vi "Boiler.vi"() -> ()   [LabVIEW 2014]
uses:
  Controls/Boiler Controls.ctl
  Controls/Boiler Simulation Controls.ctl
  Controls/Boiler Status Indicators.ctl
  Controls/Boiler state enum.ctl
  Controls/Boiler runtime status indicators.ctl
  Controls/Log file FGV action enum.ctl
  Controls/Log event enum.ctl
panel:
  in  "stop":bool
  out "Boiler Status Indicators":T1 {"Time Count" format="%.2g"}
  in  "Boiler Simulation Controls":T2 {"Flame Sensor Value (%)" min=0.0 max=100.0 scale=0.0..100.0}
  in  "Boiler Controls":T3 {"Fuel Valve Position" min=0.0 max=100.0 scale=0.0..100.0 scale format="%.2f"}
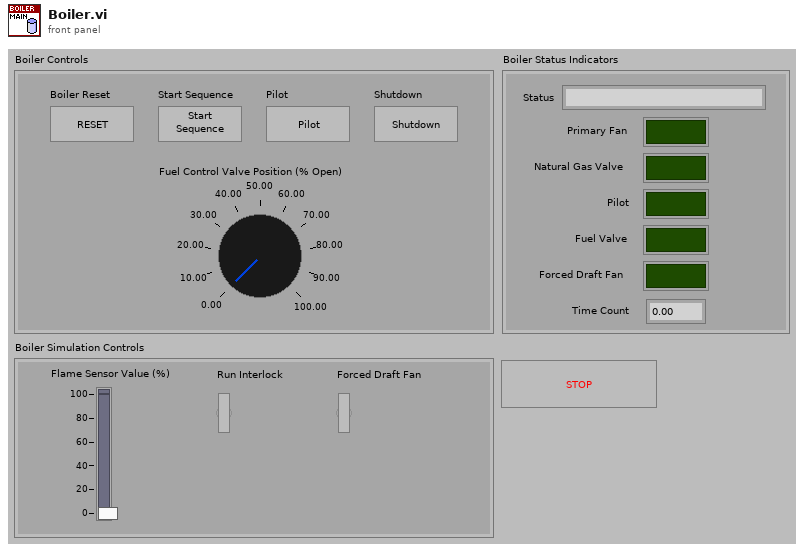
[diagram p1: front panel]
types:
  T1 = typedef "Boiler Status Indicators.ctl" = cluster{"Status":string, "Primary Fan":bool, "Natural Gas Valve":bool, "Pilot":bool, "Fuel Valve":bool, "Forced Draft Fan":bool, "Time Count":dbl}
  T2 = typedef "Boiler Simulation Controls.ctl" = cluster{"Flame Sensor Value (%)":dbl, "Run Interlock":bool, "Forced Draft Fan":bool}
  T3 = typedef "Boiler Controls.ctl" = cluster{"Boiler Reset":bool, "Start Sequence":bool, "Pilot":bool, "Shutdown":bool, "Fuel Valve Position":dbl}
  T4 = typedef "Boiler state enum.ctl" = enum16{"Initialize", "Wait on user action", "Start", "Pre-purge (running)", "Pre-purge (complete)", "Ignition (Ignite Pilot)", "Prove The Pilot", "Boiler Running", "Shutdown and Purge", "End"}
  T5 = typedef "Log file FGV action enum.ctl" = enum16{"open log file", "log event", "close log file"}
  T6 = typedef "Log event enum.ctl" = enum16{"Boiler Initialized", "Boiler Ready", "Start Pre-Purge", "Pre-Purge Complete", "Pilot ON", "Pilot proved", "Forced Draft Fan ON", "Boiler Running", "Start Shutdown Purge", "Shutdown Purge Complete"}
  T7 = typedef "Boiler runtime status indicators.ctl" = cluster{"Pre purge ready":bool, "Pre-purge complete":bool, "Pre-purge running":bool, "Pilot ignition running":bool, "Boiler Running":bool, "Shutdown running":bool, "Pilot proved":bool, "start time (ms)":u32}
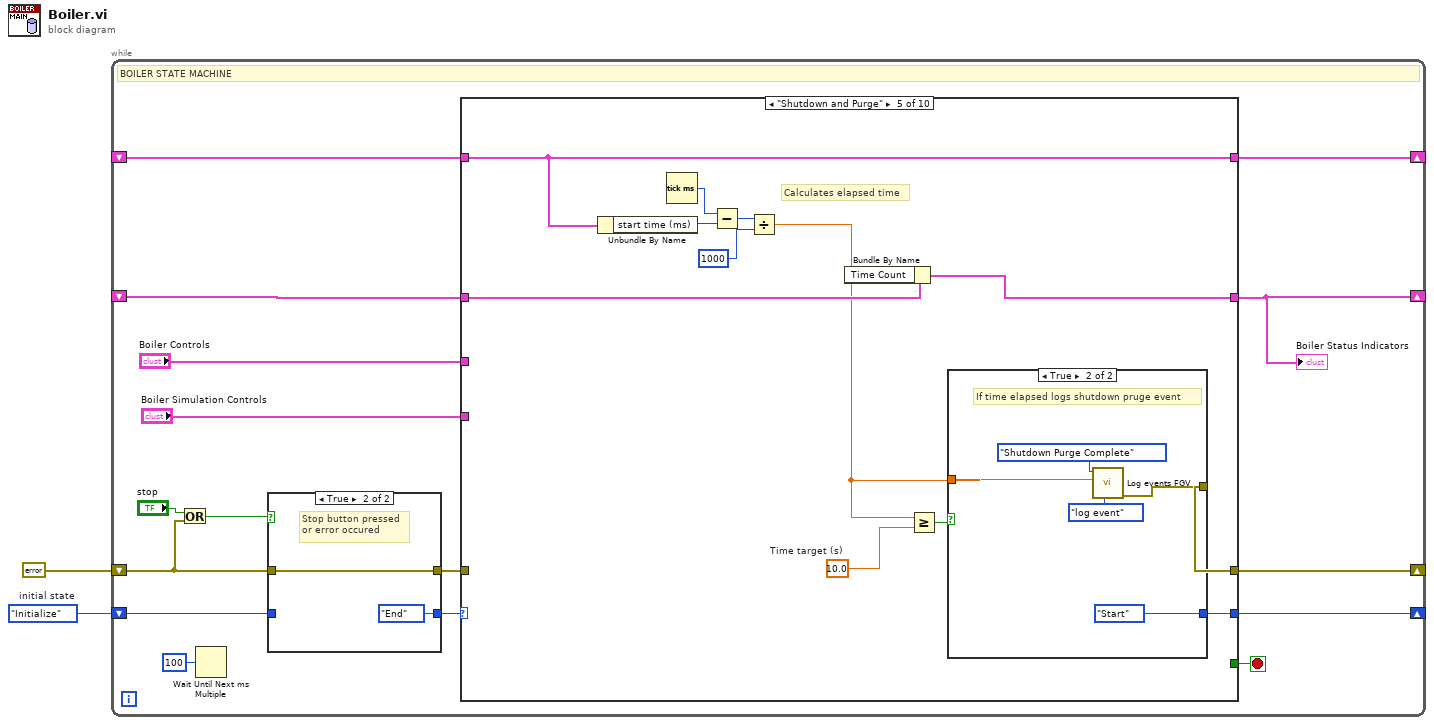
[diagram p0: block diagram]
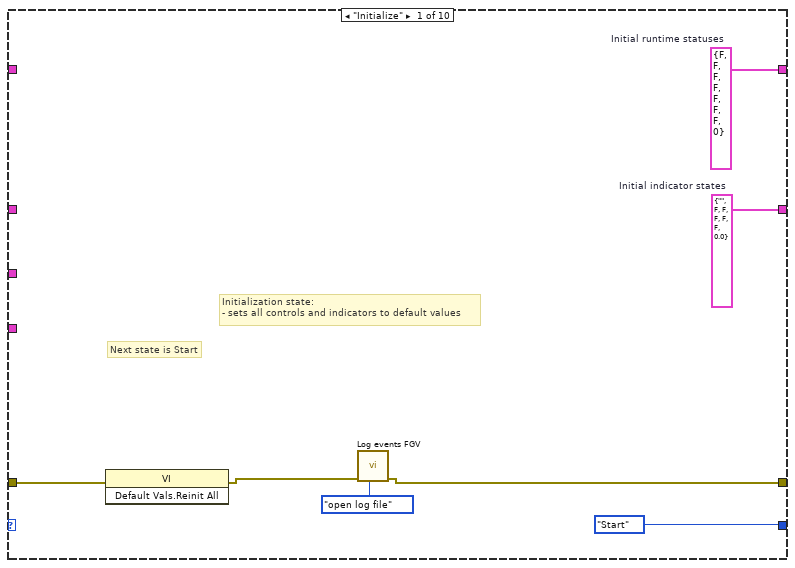
[diagram p3: hidden frame]
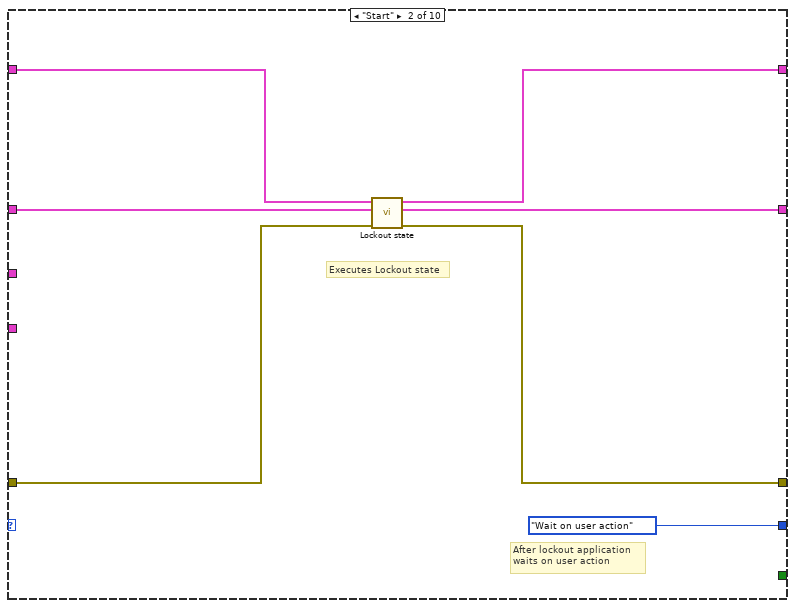
[diagram p4: hidden frame]
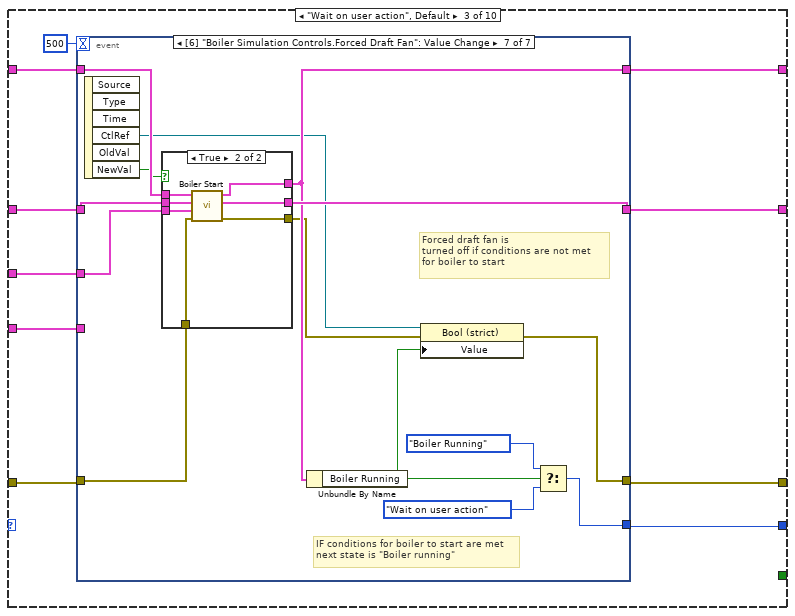
[diagram p5: hidden frame]
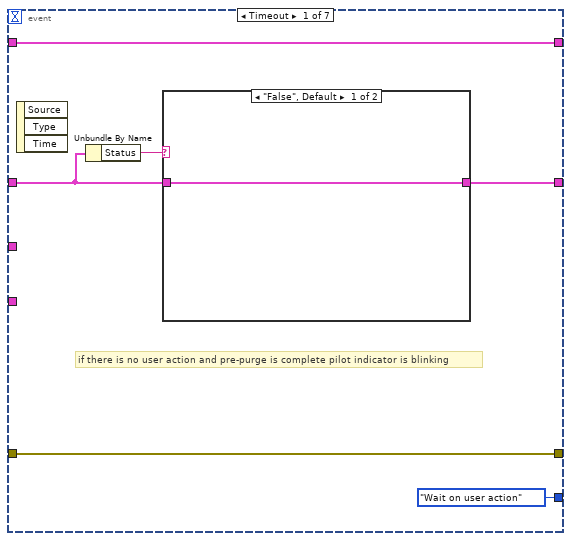
[diagram p6: hidden frame]
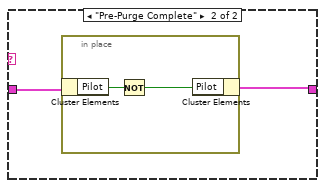
[diagram p7: hidden frame]
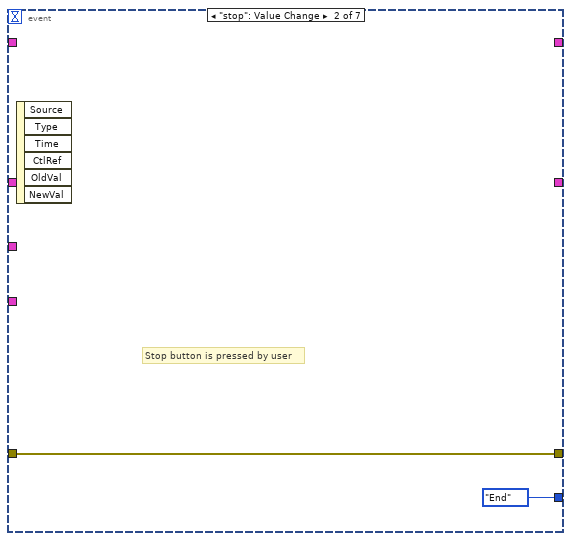
[diagram p8: hidden frame]
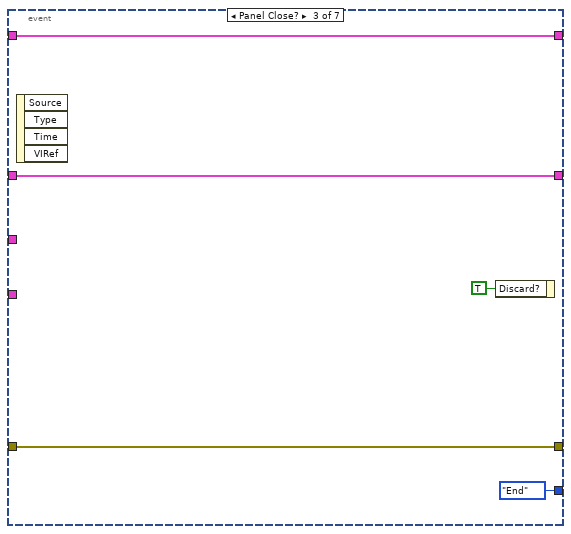
[diagram p9: hidden frame]
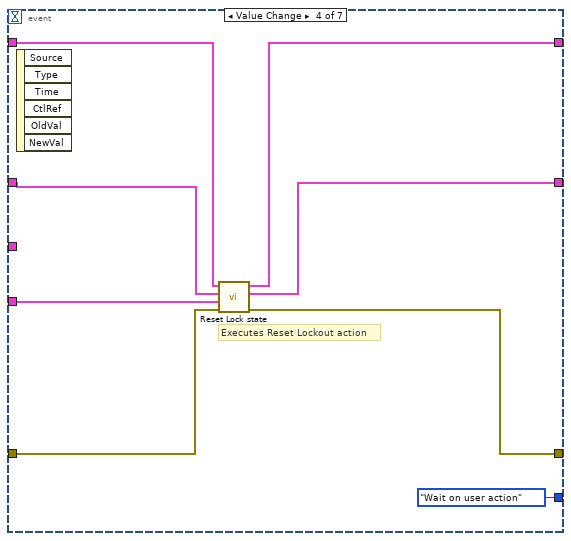
[diagram p10: hidden frame]
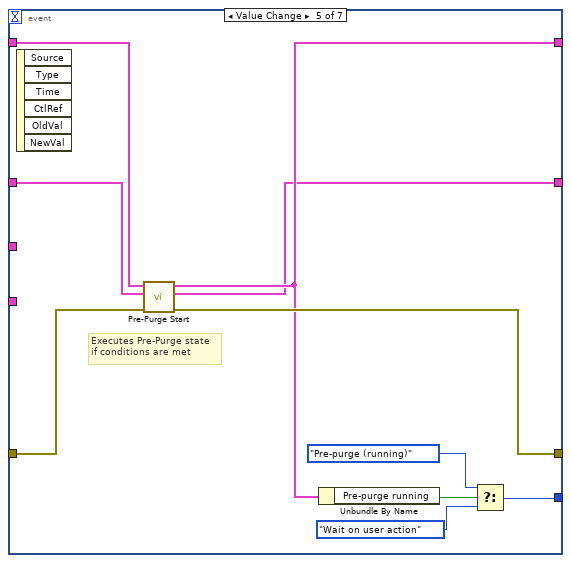
[diagram p11: hidden frame]
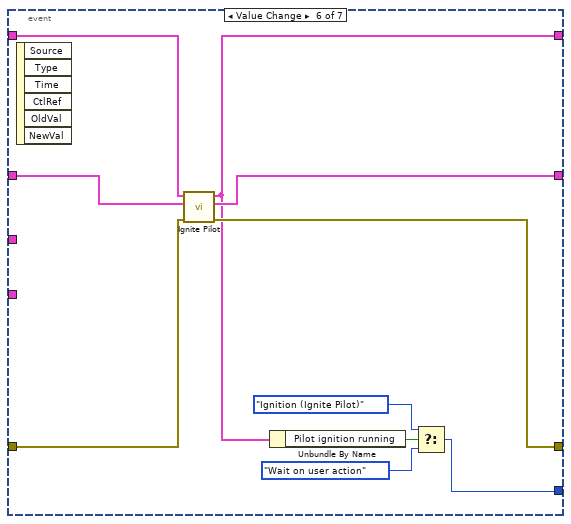
[diagram p12: hidden frame]
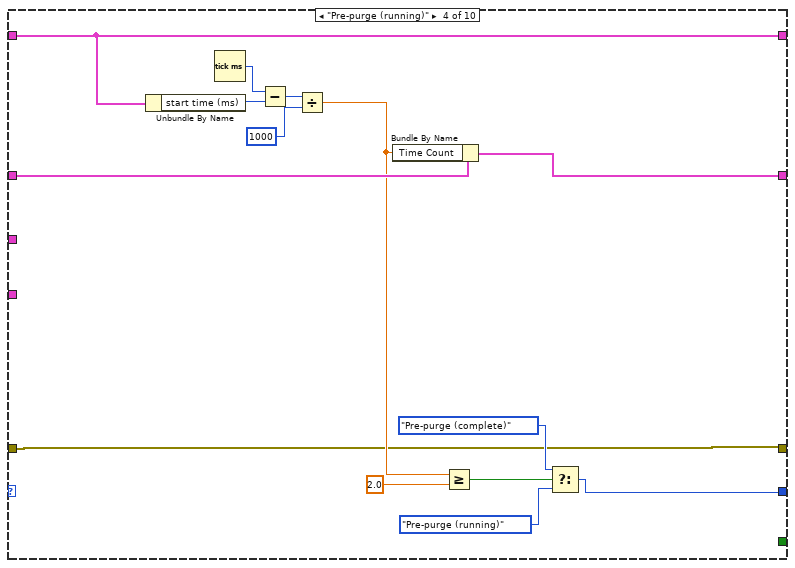
[diagram p14: hidden frame]
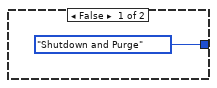
[diagram p15: hidden frame]
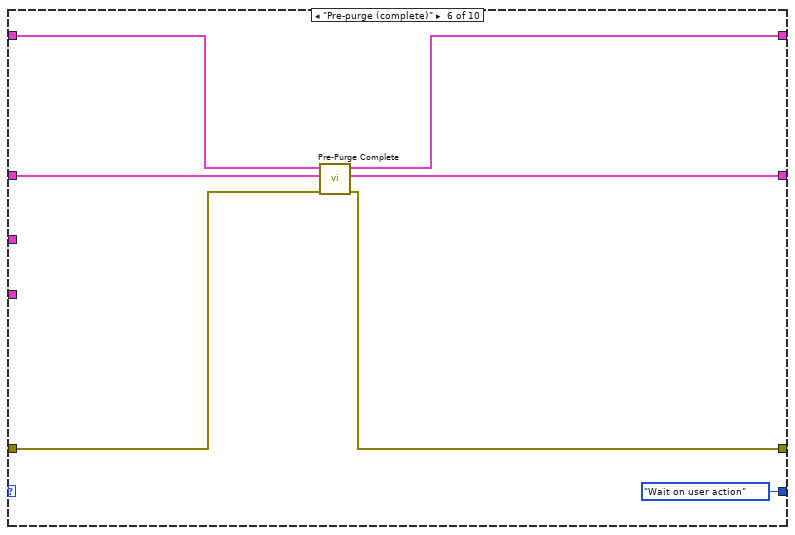
[diagram p16: hidden frame]
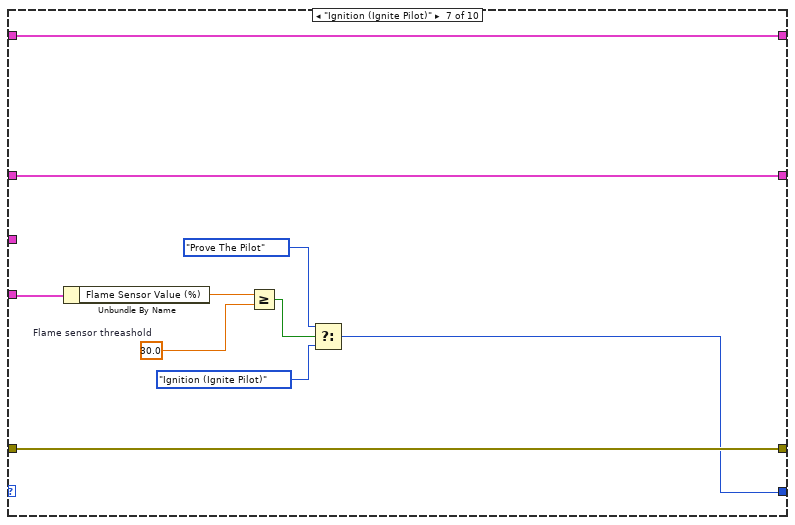
[diagram p17: hidden frame]
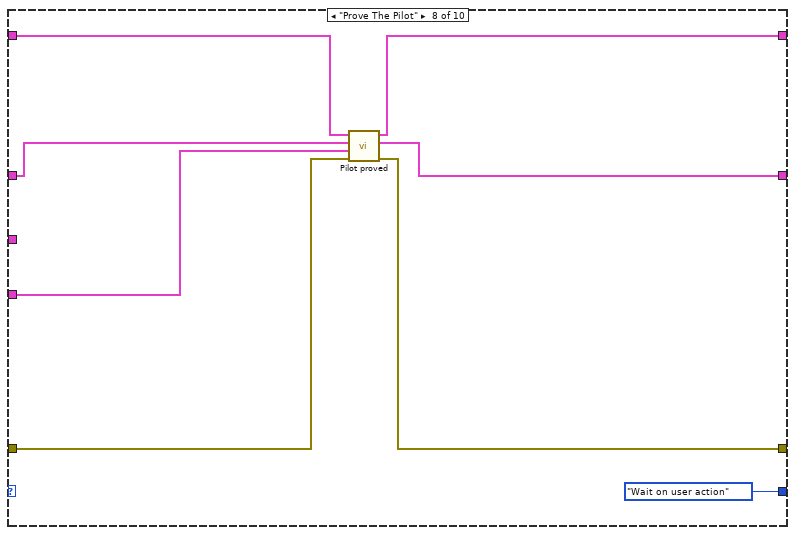
[diagram p18: hidden frame]
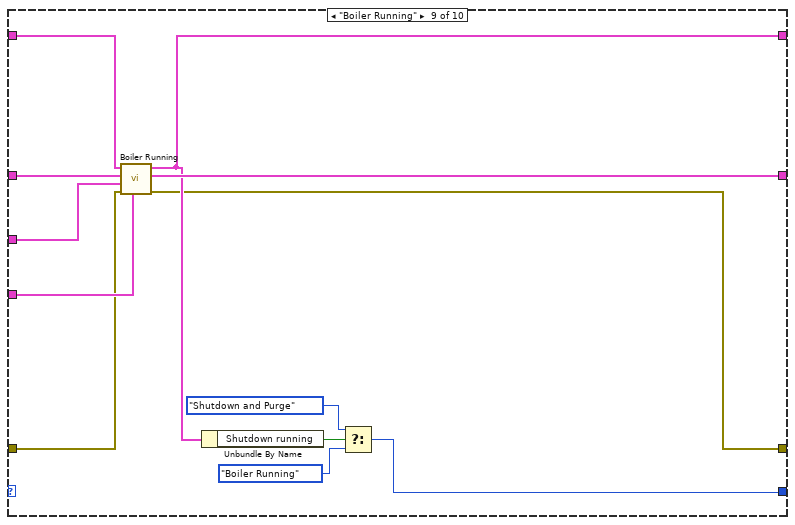
[diagram p19: hidden frame]
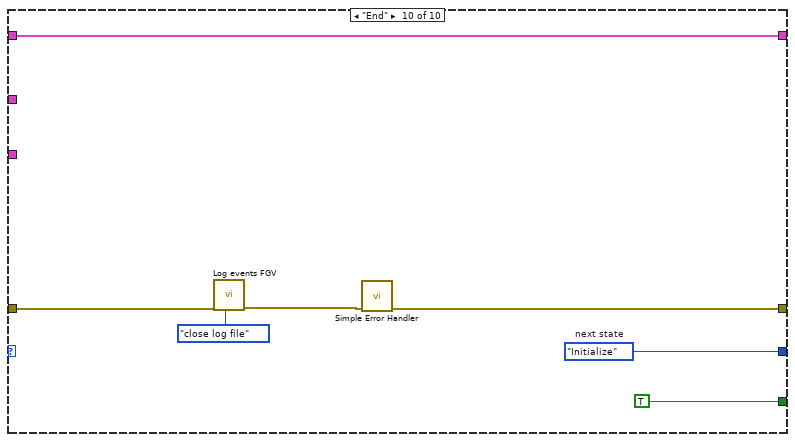
[diagram p20: hidden frame]
diagram:
  w2 = Boiler_state_enum."Initialize"  # initial state
  n1 = while {
    shift-right: [w8] -> _
    shift-left: w2 -> [w13]
    shift-right: [w17] -> _
    shift-left: _ -> [w18]
    shift-right: [w10] -> _
    shift-left: errorcluster {"status"=FALSE, "code"=0, "source"=""} ("error constant") -> [w12]
    shift-right: [w6] -> _
    shift-left: _ -> [w7]
    stop <- w9 stop-if-true
    # "BOILER STATE MACHINE"
    n2 = Or(x="stop", y=w12) -> (x .or. y?=w15:bool)
    n3 = Wait Until Next ms Multiple(millisecond multiple=u32 100) -> ()  [unwired: 1 out]
    n4 = case shown="True" w15 {
      tunnel: [w20 Boiler_state_enum."End" ("initial state")] -> w14
      tunnel: w13 -> [w20 _]
      tunnel: w12 -> [w19 w21]
      tunnel: [w19 w21] -> w11
      frame False {
      }
      frame True {
        # "Stop button pressed\nor error occured"
      }
    }
    n5 = case shown="\"Shutdown and Purge\"" w14 {
      tunnel: [w26 w32 w41 w124 w136 w151 w164 w168 w183 w190] -> w17
      tunnel: w18 -> [_ w33 w42 w125 w137 w154 w164 w169 w184 w190]
      tunnel: w11 -> [w29 w36 w45 w117 _ w155 w163 w173 w180 w187]
      tunnel: [w24 w35 w40 w117 w132 w149 w163 w172 w177 w189] -> w10
      tunnel: [_ _ _ _ _ _ _ _ _ TRUE] -> w9
      tunnel: [Boiler_state_enum."Start" ("initial state") Boiler_state_enum."Wait on user action" ("next state") w46 w120 w131 Boiler_state_enum."Wait on user action" ("next state") w157 Boiler_state_enum."Wait on user action" ("next state") w174 w191] -> w8
      tunnel: w7 -> [_ w31 w44 w130 w142 w153 w165 w171 w185 _]
      tunnel: [w27 w30 w43 w130 w142 w152 w165 w170 w179 _] -> w6
      tunnel: "Boiler Simulation Controls" -> [_ _ w37 _ _ _ w162 w166 w181 _]
      tunnel: "Boiler Controls" -> [_ _ w38 _ _ _ _ _ w182 _]
      frame "Initialize" {
        w26 = T1 {"Status"="", "Primary Fan"=FALSE, "Natural Gas Valve"=FALSE, "Pilot"=FALSE, "Fuel Valve"=FALSE, "Forced Draft Fan"=FALSE, "Time Count"=0.0}  # Initial indicator states
        w27 = T7 {"Pre purge ready"=FALSE, "Pre-purge complete"=FALSE, "Pre-purge running"=FALSE, "Pilot ignition running"=FALSE, "Boiler Running"=FALSE, "Shutdown running"=FALSE, "Pilot proved"=FALSE, "start time (ms)"=0}  # Initial runtime statuses
        # "Next state is Start"
        # "Initialization state:\n- sets all controls and indicators to default values"
        n6 = invoke class="VI" method="Default Vals.Reinit All"(error in=w29) -> (error out=w25:errorcluster)  [unwired: 2 in, 2 out]
        n7 = call "Log events FGV.vi"("action"=Log_file_FGV_action_enum."open log file", "error in (no error)"=w25) -> ("error out"=w24:errorcluster)  [unwired: 9 in]
      }
      frame "Start" {
        # "After lockout application\nwaits on user action"
        # "Executes Lockout state"
        n8 = call "Lockout state.vi"("error in (no error)"=w36, "Initial indicator states in"=w33, "Runtime statuses in"=w31) -> ("error out"=w35:errorcluster, "Initial indicator states out"=w32:T1, "Runtime statuses out"=w30:T7)  [unwired: 6 in]
      }
      frame "Wait on user action", Default {
        n9 = event shown="[6] \"Boiler Simulation Controls.Forced Draft Fan\": Value Change" {
          selector: _ -> [_ _ _ _ _ _ _]
          dyn-events: _ -> [_ _ _ _ _ _ _]
          timeout: 500 -> [_ _ _ _ _ _ _]
          tunnel: [Boiler_state_enum."Wait on user action" ("initial state") Boiler_state_enum."End" ("initial state") Boiler_state_enum."End" ("initial state") Boiler_state_enum."Wait on user action" ("initial state") w74 w83 w99] -> w46
          tunnel: [w51 w58 w61 w71 w81 w88 w96] -> w40
          tunnel: w45 -> [w51 w58 w61 w72 w82 w90 w103]
          tunnel: w44 -> [w52 _ w63 w69 w78 w92 w106]
          tunnel: [w52 _ w63 w68 w80 w87 w100] -> w43
          tunnel: w42 -> [w47 _ w62 w67 w77 w91 w104]
          tunnel: [w48 _ w62 w66 w79 w89 w105] -> w41
          tunnel: w38 -> [_ _ _ _ _ _ w98]
          tunnel: w37 -> [_ _ _ w65 _ _ _]
          event Timeout {
            # "if there is no user action and pre-purge is complete pilot indicator is blinking"
            n10 = event-data() -> ()  [unwired: 1 in, 3 out]
            n11 = Unbundle By Name(w47) -> ("Status"=w49:string)
            n12 = case shown="\"False\", Default" w49 {
              tunnel: [w53 w54] -> w48
              tunnel: w47 -> [w53 w55]
              frame "False", Default {
              }
              frame "Pre-Purge Complete" {
                n13 = in-place {
                  n14 = in-place-cluster #1(w55) -> ("Pilot"=w57:bool)
                  n15 = Not(x=w57) -> (.not. x?=w56:bool)
                  n16 = in-place-cluster #1("Pilot"=w56) -> (w54:T1)
                }
              }
            }
          }
          event "stop": Value Change {
            # "Stop button is pressed by user"
            n17 = event-data() -> ()  [unwired: 1 in, 6 out]
          }
          event Panel Close? {
            n18 = event-data() -> ()  [unwired: 1 in, 4 out]
            n19 = event-data("Discard?"=TRUE) -> ()  [unwired: 1 in, 1 out]
          }
          event Value Change {
            # "Executes Reset Lockout action"
            n20 = event-data() -> ()  [unwired: 1 in, 6 out]
            n21 = call "Reset Lock state.vi"("error in (no error)"=w72, "Boiler Simulation Controls"=w65, "Indicator states in"=w67, "Runtime statuses in"=w69) -> ("error out"=w71:errorcluster, "Indicator states out"=w66:T1, "Runtime statuses out"=w68:T7)  [unwired: 5 in]
          }
          event Value Change {
            # "Executes Pre-Purge state\nif conditions are met"
            n22 = event-data() -> ()  [unwired: 1 in, 6 out]
            n23 = call "Pre-Purge Start.vi"("error in (no error)"=w82, "Indicator states in"=w77, "Runtime statuses in"=w78) -> ("error out"=w81:errorcluster, "Indicator states out"=w79:T1, "Runtime statuses out"=w80:T7)  [unwired: 6 in]
            n24 = Unbundle By Name(w80) -> ("Pre-purge running"=w76:bool)
            n25 = Select(t=Boiler_state_enum."Pre-purge (running)" ("initial state"), s=w76, f=Boiler_state_enum."Wait on user action" ("initial state")) -> (s? t:f=w74:T4)
          }
          event Value Change {
            n26 = event-data() -> ()  [unwired: 1 in, 6 out]
            n27 = call "Ignite Pilot.vi"("error in (no error)"=w90, "Indicator states in"=w91, "Runtime statuses in"=w92) -> ("error out"=w88:errorcluster, "Indicator states out"=w89:T1, "Runtime statuses out"=w87:T7)  [unwired: 6 in]
            n28 = Unbundle By Name(w87) -> ("Pilot ignition running"=w86:bool)
            n29 = Select(t=Boiler_state_enum."Ignition (Ignite Pilot)" ("initial state"), s=w86, f=Boiler_state_enum."Wait on user action" ("initial state")) -> (s? t:f=w83:T4)
          }
          event Value Change {
            # "IF conditions for boiler to start are met\nnext state is \"Boiler running\""
            # "Forced draft fan is\nturned off if conditions are not met\nfor boiler to start"
            n30 = event-data() -> ("CtlRef"=w95:refnum<vi>, "NewVal"=w93:bool)  [unwired: 1 in, 4 out]
            n31 = case shown="True" w93 {
              tunnel: w106 -> [w109 w116]
              tunnel: [w108 w115] -> w105
              tunnel: w104 -> [w108 w114]
              tunnel: w103 -> [w107 w113]
              tunnel: [w109 w112] -> w100
              tunnel: w98 -> [_ w111]
              tunnel: [w107 w110] -> w97
              frame False {
                # "ignores\nforced\ndraft fan\noff event"
              }
              frame True {
                n32 = call "Boiler Start.vi"("error in (no error)"=w113, "Boiler Controls"=w111, "Indicator states in"=w114, "Runtime statuses in"=w116) -> ("error out"=w110:errorcluster, "Indicator states out"=w115:T1, "Runtime statuses out"=w112:T7)  [unwired: 5 in]
              }
            }
            n33 = Unbundle By Name(w100) -> ("Boiler Running"=w94:bool)
            n34 = property class="Bool (strict)"(reference=w95, error in=w97, "Value"=w94) -> (error out=w96:errorcluster)  [unwired: 1 out]
            n35 = Select(t=Boiler_state_enum."Boiler Running" ("initial state"), s=w94, f=Boiler_state_enum."Wait on user action" ("initial state")) -> (s? t:f=w99:T4)
          }
        }
      }
      frame "Pre-purge (running)" {
        n36 = Unbundle By Name(w130) -> ("start time (ms)"=w129:u32)
        n37 = Tick Count (ms)() -> (millisecond timer value=w128:u32)
        n38 = Subtract(x=w128, y=w129) -> (x-y=w127:u32)
        n39 = Divide(x=w127, y=u32 1000) -> (x/y=w118:dbl)
        n40 = Bundle By Name(cluster=w125, "Time Count"=w118) -> (w124:T1)
        n41 = Greater Or Equal?(x=w118, y=2.0) -> (x >= y?=w122:bool)
        n42 = Select(t=Boiler_state_enum."Pre-purge (complete)" ("next state"), s=w122, f=Boiler_state_enum."Pre-purge (running)" ("next state")) -> (s? t:f=w120:T4)
      }
      frame "Shutdown and Purge" {
        w135 = 10.0  # Time target (s)
        # "Calculates elapsed time"
        n43 = Unbundle By Name(w142) -> ("start time (ms)"=w141:u32)
        n44 = Tick Count (ms)() -> (millisecond timer value=w140:u32)
        n45 = Subtract(x=w140, y=w141) -> (x-y=w139:u32)
        n46 = Divide(x=w139, y=u32 1000) -> (x/y=w133:dbl)
        n47 = Bundle By Name(cluster=w137, "Time Count"=w133) -> (w136:T1)
        n48 = Greater Or Equal?(x=w133, y=w135) -> (x >= y?=w134:bool)
        n49 = case shown="True" w134 {
          tunnel: w133 -> [_ w146]
          tunnel: [_ w145] -> w132
          tunnel: [Boiler_state_enum."Shutdown and Purge" ("next state") Boiler_state_enum."Start" ("next state")] -> w131
          frame False {
          }
          frame True {
            # "If time elapsed logs shutdown pruge event"
            n50 = call "Log events FGV.vi"("action"=Log_file_FGV_action_enum."log event", "Event data"=w146, "Log event"=Log_event_enum."Shutdown Purge Complete") -> ("error out"=w145:errorcluster)  [unwired: 8 in]
          }
        }
      }
      frame "Pre-purge (complete)" {
        n51 = call "Pre-Purge Complete.vi"("error in (no error)"=w155, "Indicator states in"=w154, "Runtime statuses in"=w153) -> ("error out"=w149:errorcluster, "Indicator states out"=w151:T1, "Runtime statuses out"=w152:T7)  [unwired: 6 in]
      }
      frame "Ignition (Ignite Pilot)" {
        w156 = 30.0  # Flame sensor threashold
        n52 = Unbundle By Name(w162) -> ("Flame Sensor Value (%)"=w161:dbl)
        n53 = Greater Or Equal?(x=w161, y=w156) -> (x >= y?=w160:bool)
        n54 = Select(t=Boiler_state_enum."Prove The Pilot" ("next state"), s=w160, f=Boiler_state_enum."Ignition (Ignite Pilot)" ("next state")) -> (s? t:f=w157:T4)
      }
      frame "Prove The Pilot" {
        n55 = call "Pilot proved.vi"("error in (no error)"=w173, "Boiler Simulation Controls"=w166, "Indicator states in"=w169, "Runtime statuses in"=w171) -> ("error out"=w172:errorcluster, "Indicator states out"=w168:T1, "Runtime statuses out"=w170:T7)  [unwired: 5 in]
      }
      frame "Boiler Running" {
        n56 = call "Boiler Running.vi"("Boiler Simulation Controls"=w181, "error in (no error)"=w180, "Boiler Controls"=w182, "Indicator states in"=w184, "Runtime statuses in"=w185) -> ("error out"=w177:errorcluster, "Indicator states out"=w183:T1, "Runtime statuses out"=w179:T7)  [unwired: 4 in]
        n57 = Unbundle By Name(w179) -> ("Shutdown running"=w178:bool)
        n58 = Select(t=Boiler_state_enum."Shutdown and Purge" ("next state"), s=w178, f=Boiler_state_enum."Boiler Running" ("next state")) -> (s? t:f=w174:T4)
      }
      frame "End" {
        w191 = Boiler_state_enum."Initialize"  # next state
        n59 = call "Log events FGV.vi"("action"=Log_file_FGV_action_enum."close log file", "error in (no error)"=w187) -> ("error out"=w186:errorcluster)  [unwired: 9 in]
        n60 = call <vilib>:"Simple Error Handler.vi"("error in (no error)"=w186) -> ("error out"=w189:errorcluster)  [unwired: 4 in, 4 out]
      }
    }
    "Boiler Status Indicators" <- w17
  }
